vi "Control system.vi"() -> ()   [LabVIEW 2019]
panel:
  out "УЗ5":dbl
  out "Насос 8":bool=TRUE
  out "КР1":dbl
  out "КР7":dbl
  out "КР5":dbl
  out "КР3":dbl
  out "КР8":dbl
  out "КР4":dbl
  out "КР6":dbl
  out "КР2":dbl
  out "УЗ5":dbl
  out "УЗ7":dbl
  out "УЗ6":dbl
  out "СЧ2":dbl
  out "Манометр":dbl
  out "Насос 4":bool=TRUE
  out "ДМ2":dbl
  out "УЗ5":dbl
  out "Насос 3":bool=TRUE
  out "СЧ1":dbl
  out "УЗ2":dbl
  out "ДМ1":dbl
  out "УЗ3":dbl
  out "Объем подачи ДН2":dbl format="%#_13g"
  out "Донный клапан":bool=TRUE
  out "Дозирующий насос 2":bool=TRUE
  out "Насос 2":bool=TRUE
  out "PH1":dbl
  out "Насос 1":bool=TRUE
  out "УЗ2":dbl
  out "ДН1 объем подачи":dbl format="%#_13g"
  out "УЗ1":dbl
  out "Дозирующий насос 1":bool=TRUE
  out "УЗ4":dbl
  in  "Насос 8":bool=TRUE
  in  "КР1":dbl
  in  "КР8":dbl
  in  "КР4":dbl
  in  "КР7":dbl
  in  "КР6":dbl
  in  "КР5":dbl
  in  "КР3":dbl
  in  "КР2":dbl
  in  "Насос 4":bool=TRUE
  in  "Насос 3":bool=TRUE
  in  "объем подачи ДН2":dbl format="%#_13g"
  in  "Донный клапан":bool=TRUE
  in  "Дозирующий насос 2":bool=TRUE
  in  "Насос 2":bool=TRUE
  in  "ДН1 объем подачи":dbl format="%#_13g"
  in  "Дозирующий насос 1":bool=TRUE
  in  "Насос 1":bool=TRUE
  out "Статус работы":string
  in  "stop":bool
  # "Индикаторы промывки"
  # "Меабрана"
  # "Биореактор"
  # "II ступень очистки"
  # "I ступень очистки"
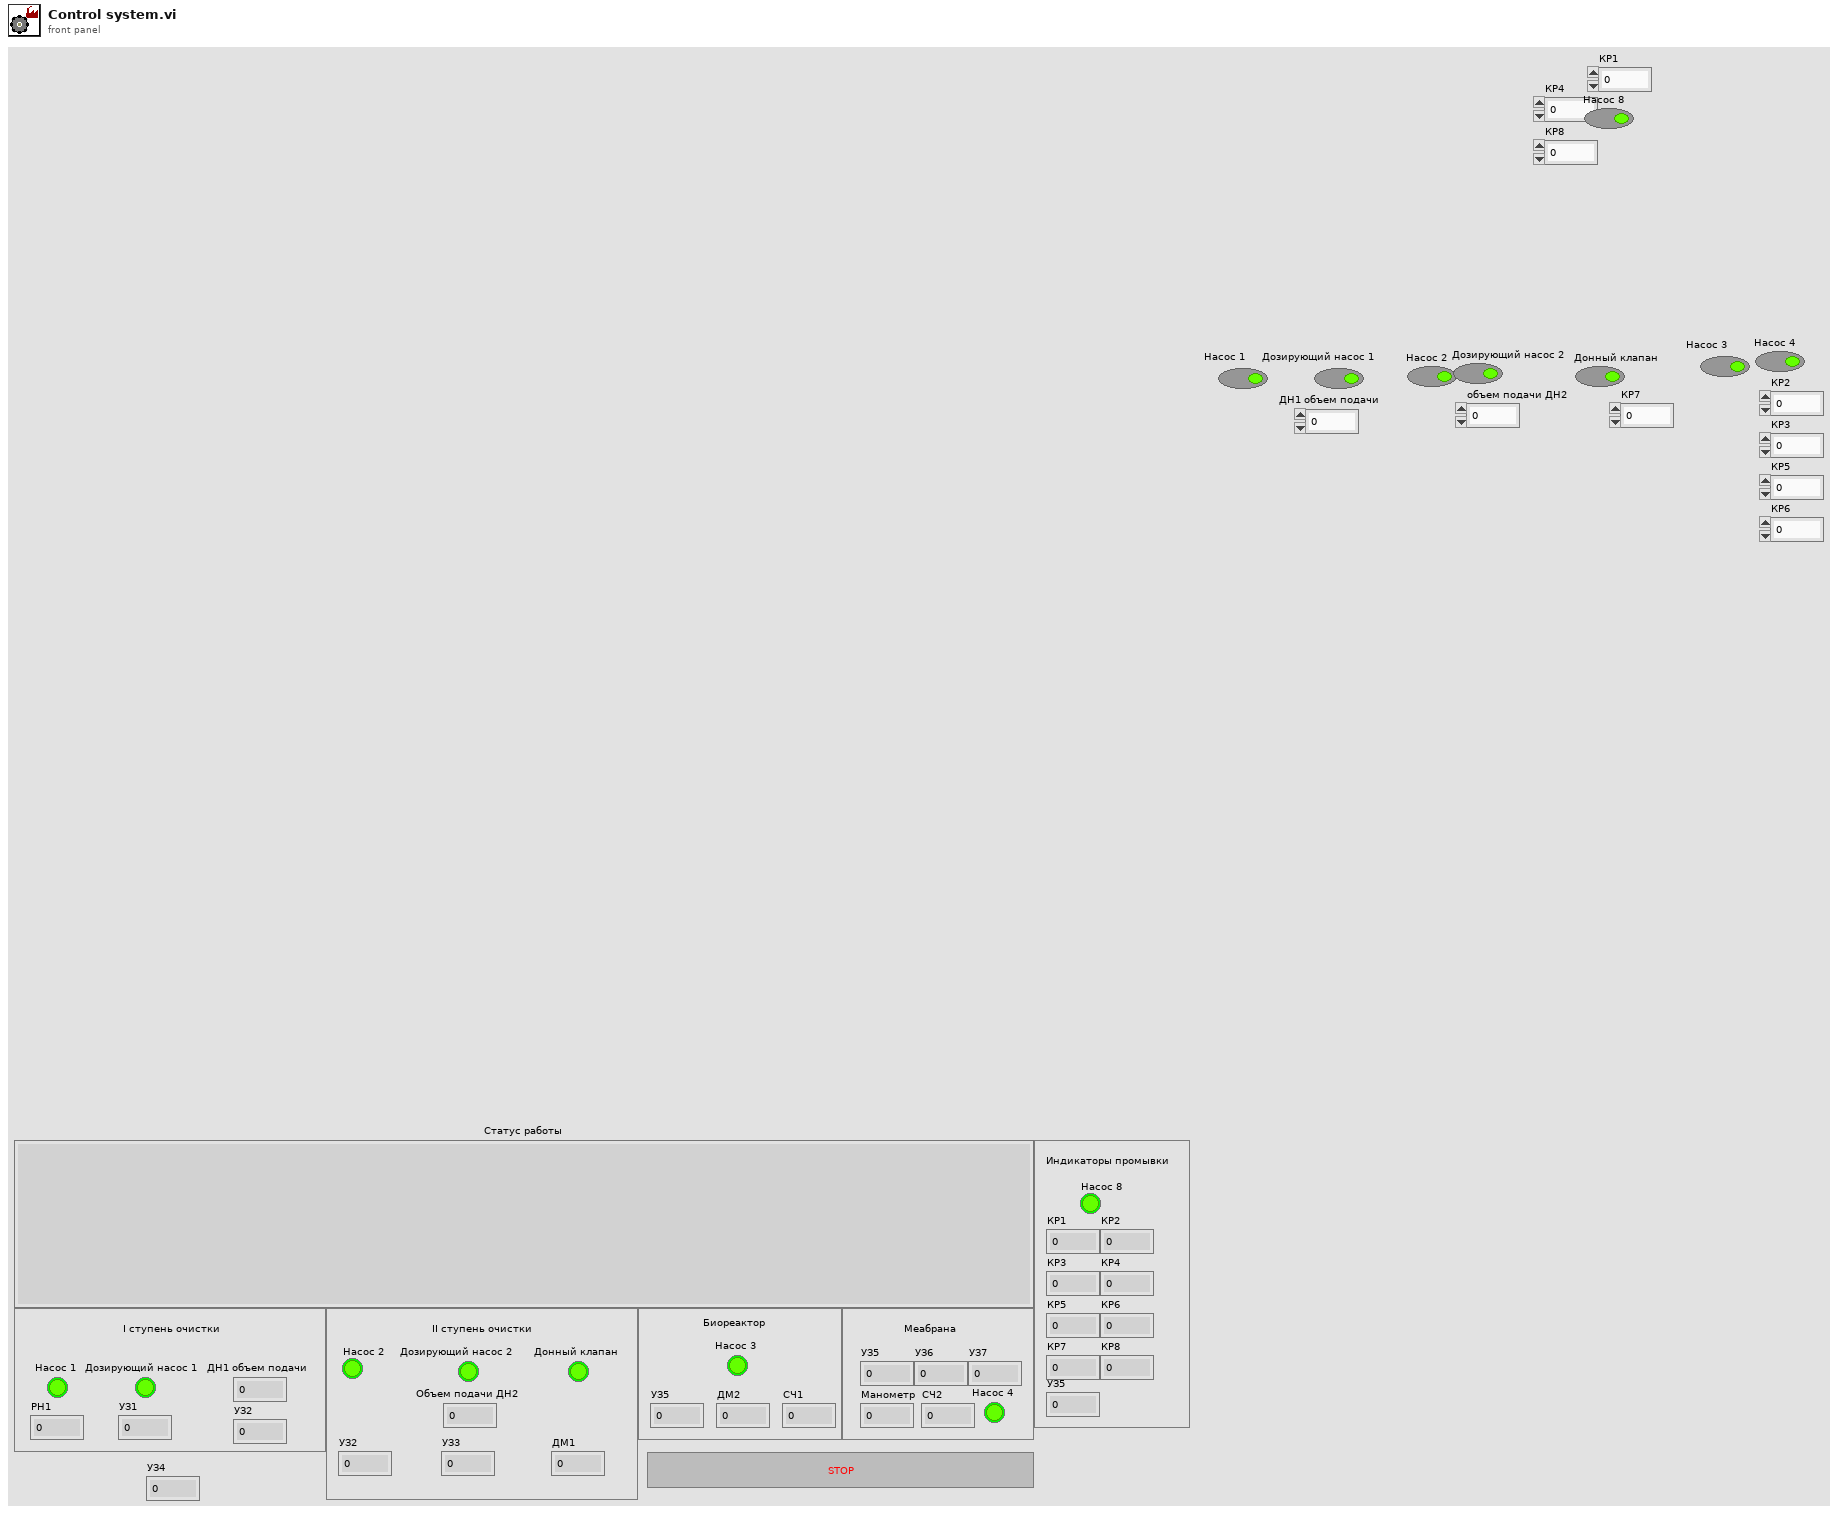
[diagram p1: front panel]
types:
  T1 = cluster{"УЗ1":dbl, "УЗ2":dbl, "УЗ3":dbl, "УЗ4":dbl, "УЗ5":dbl, "УЗ6":dbl, "УЗ7":dbl, "PH1":dbl, "ДМ1":dbl, "ДМ2":dbl, "Манометр":dbl, " СЧ1":dbl, " СЧ2":dbl}
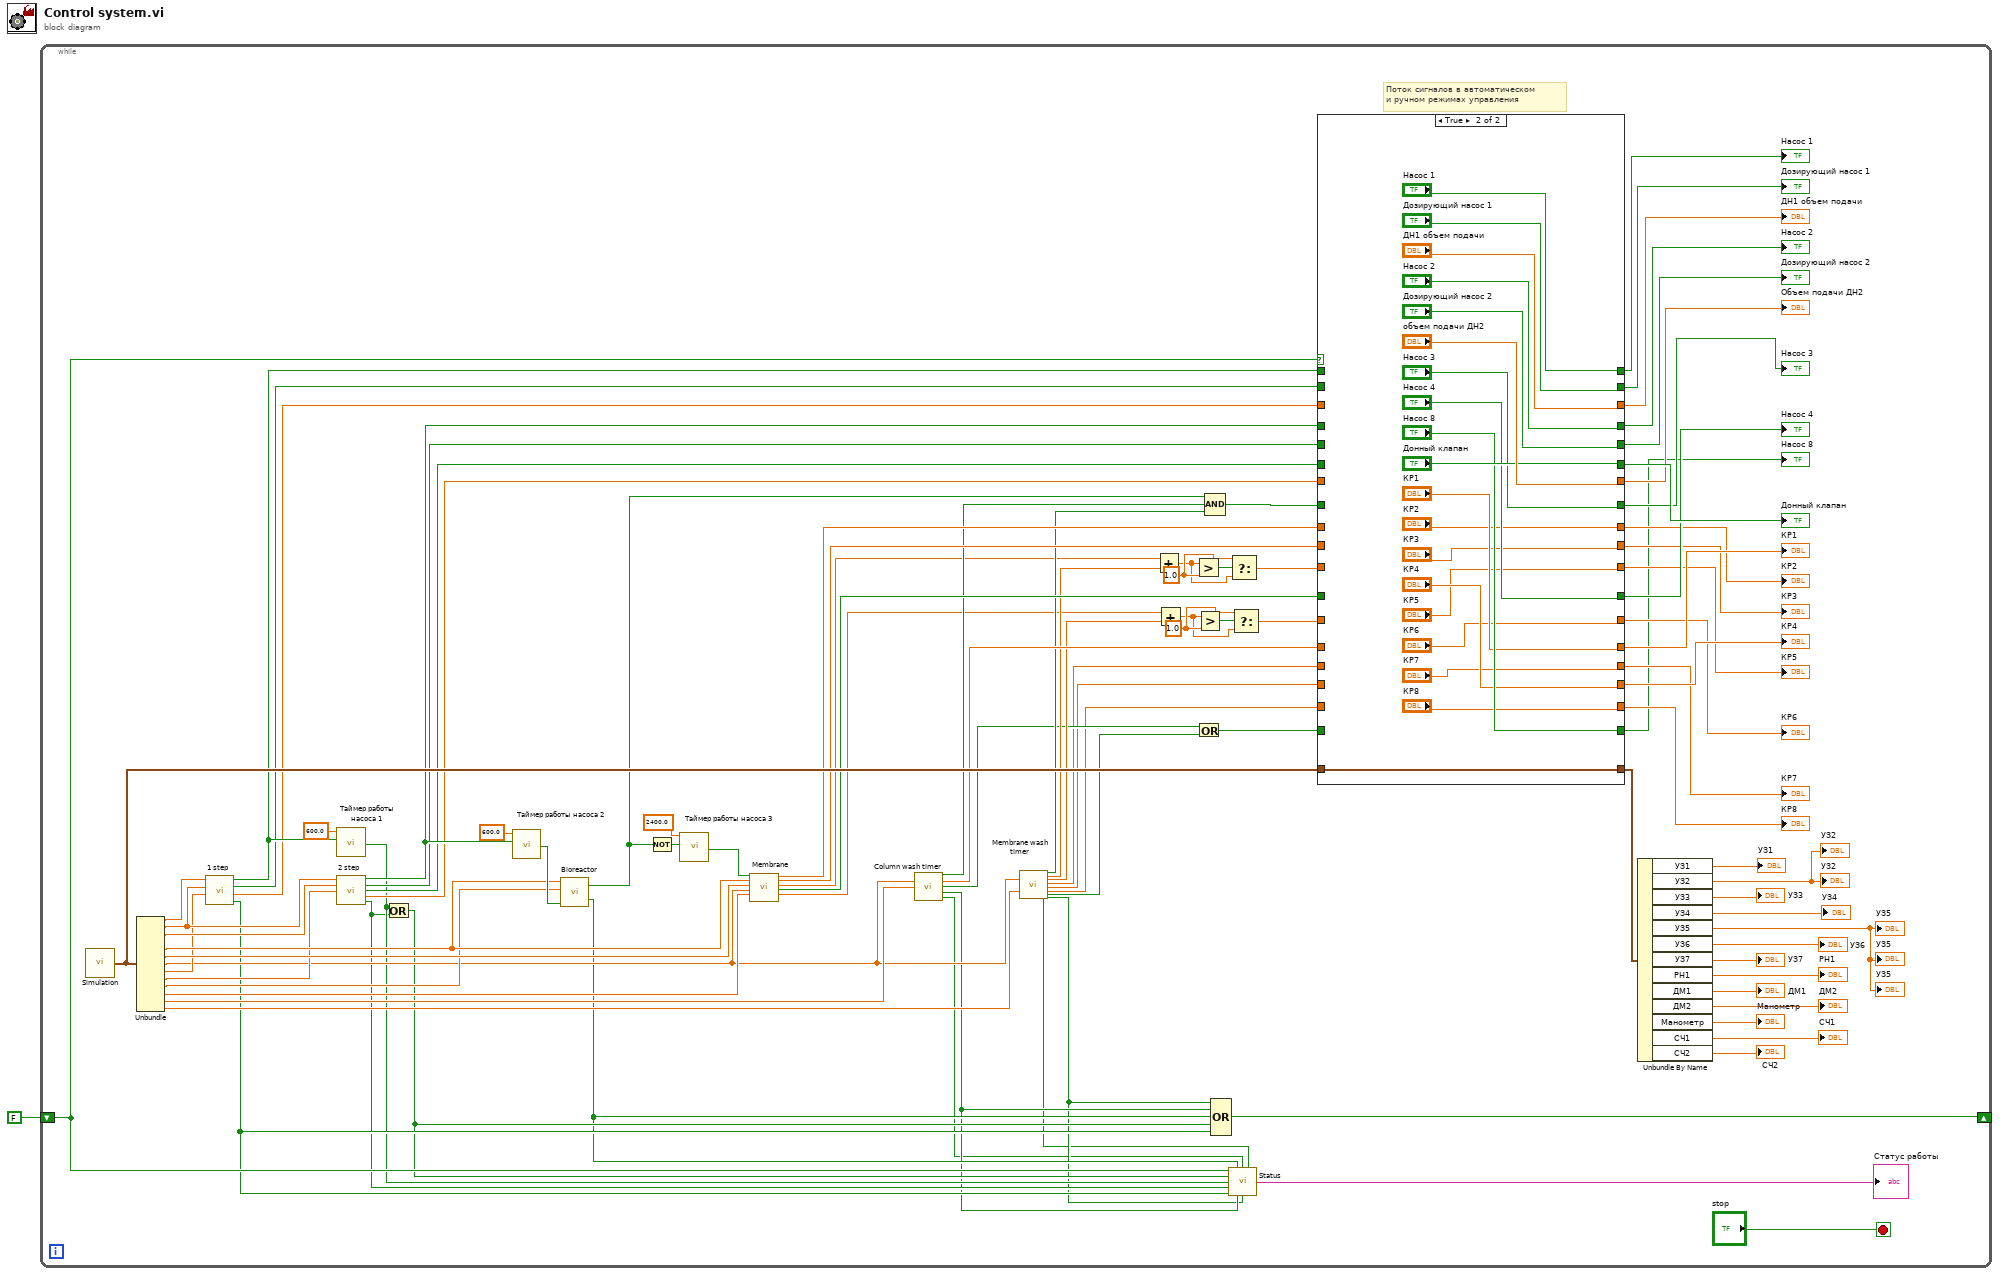
[diagram p0: block diagram]
diagram:
  n1 = while {
    shift-right: [w82] -> _
    shift-left: FALSE ("Error output") -> [w26]
    stop <- "stop" stop-if-true
    w55 = 1.0 ("y")
    w59 = 1.0 ("y")
    # "Поток сигналов в автоматическом \nи ручном режимах управления"
    n2 = call "Simulation.vi"() -> ("output cluster"=w80:T1)
    n3 = Unbundle(w80) -> ("УЗ1"=w92:dbl, "УЗ2"=w91:dbl, "УЗ3"=w90:dbl, "УЗ5"=w88:dbl, "УЗ6"=w89:dbl, "УЗ7"=w65:dbl, "PH1"=w87:dbl, "ДМ1"=w86:dbl, "ДМ2"=w85:dbl, "Манометр"=w84:dbl, "СЧ1"=w81:dbl, "СЧ2"=w64:dbl)  [unwired: 1 out]
    n4 = call "1 step.vi"("PH1"=w87, "УЗ2"=w91, "УЗ1"=w92) -> ("Error output"=w25:bool, "ДН1 объем подачи"=w77:dbl, "Дозирующий насос 1"=w78:bool, "Насос 1"=w79:bool)  [unwired: 1 in]
    n5 = call "Таймер работы насоса 1"("Time Target (s)"=600.0, "Reset"=w79) -> ("Time has Elapsed"=w23:bool)  [unwired: 10 in, 7 out]
    n6 = call "2 step.vi"("УЗ2"=w91, "УЗ3"=w90, "ДМ1"=w86) -> ("Насос 2"=w76:bool, "ДН2"=w75:bool, "Донный клапан"=w74:bool, "объем подачи ДН2"=w73:dbl, "Error output"=w22:bool)  [unwired: 8 in]
    n7 = Or(x=w23, y=w22) -> (x .or. y?=w24:bool)
    n8 = call "Таймер работы насоса 2"("Time Target (s)"=600.0, "Reset"=w76) -> ("Time has Elapsed"=w96:bool)  [unwired: 10 in, 7 out]
    n9 = call "Bioreactor.vi"("Timer"=w96, "ДМ2"=w85, "УЗ5"=w88) -> ("Error output"=w21:bool, "Насос 3"=w68:bool)  [unwired: 1 in]
    n10 = Not(x=w68) -> (.not. x?=w94:bool)
    n11 = call "Таймер работы насоса 3"("Time Target (s)"=2400.0, "Reset"=w94) -> ("Time has Elapsed"=w93:bool)  [unwired: 10 in, 7 out]
    n12 = call "Membrane.vi"("Насос 3"=w93, "УЗ5"=w88, "УЗ6"=w89, "УЗ7"=w65, "Манометр"=w84) -> ("КР2"=w72:dbl, "КР3"=w71:dbl, "КР5"=w61:dbl, "Насос 4"=w70:bool, "КР6"=w53:dbl)  [unwired: 10 in]
    n13 = call "Column wash timer.vi"("УЗ7"=w65, "СЧ1"=w81) -> ("Насос 3"=w67:bool, "КР1"=w66:dbl, "Насос 8"=w49:bool, "Error output"=w20:bool, "Status"=w17:bool)  [unwired: 9 in]
    n14 = call "Membrane wash timer.vi"("УЗ7"=w65, "СЧ2"=w64) -> ("Status"=w18:bool, "Насос 3"=w63:bool, "КР5"=w62:dbl, "КР6"=w52:dbl, "КР7"=w47:dbl, "КР4"=w46:dbl, "КР8"=w45:dbl, "Насос 8"=w48:bool, "Error output"=w19:bool)  [unwired: 17 in]
    n15 = Add(x=w61, y=w62) -> (x+y=w58:dbl)
    n16 = Add(x=w53, y=w52) -> (x+y=w54:dbl)
    n17 = Greater?(x=w58, y=w59) -> (0:w60:bool)
    n18 = Or(x=w49, y=w48) -> (x .or. y?=w50:bool)
    n19 = Greater?(x=w54, y=w55) -> (0:w56:bool)
    n20 = Compound Arithmetic op=AND(w68, w67, w63) -> (w69:bool)
    n21 = Compound Arithmetic op=OR(w19, w20, w21, w24, w25) -> (w82:bool)
    n22 = call "Status.vi"("Membrane washing status"=w18, "Column washing status"=w17, "Membrane washing error"=w19, "Bioreactor error"=w21, "Column washing error"=w20, "Error input"=w26, "2 step error"=w24, "2 step error-1"=w23, "2 step error-2"=w22, "1 step error"=w25) -> ("Status output"=→"Статус работы":string)  [unwired: 5 in]
    n23 = Select(t=w59, s=w60, f=w58) -> (s? t:f=w57:dbl)
    n24 = Select(t=w55, s=w56, f=w54) -> (s? t:f=w51:dbl)
    n25 = case shown="True" w26 {
      tunnel: w80 -> [w104 w136]
      tunnel: w79 -> [w117 _]
      tunnel: w78 -> [w116 _]
      tunnel: w77 -> [w115 _]
      tunnel: w76 -> [w114 _]
      tunnel: w75 -> [w113 _]
      tunnel: w74 -> [w112 _]
      tunnel: w73 -> [w111 _]
      tunnel: w69 -> [w110 _]
      tunnel: w72 -> [w109 _]
      tunnel: w71 -> [w108 _]
      tunnel: w57 -> [w107 _]
      tunnel: w70 -> [w106 _]
      tunnel: w51 -> [w105 _]
      tunnel: [w117 "Насос 1"] -> w44
      tunnel: [w116 "Дозирующий насос 1"] -> w43
      tunnel: [w115 "ДН1 объем подачи"] -> w42
      tunnel: [w114 "Насос 2"] -> w41
      tunnel: [w113 "Дозирующий насос 2"] -> w40
      tunnel: [w112 "Донный клапан"] -> w39
      tunnel: [w111 "объем подачи ДН2"] -> w38
      tunnel: [w110 "Насос 3"] -> w37
      tunnel: [w109 "КР2"] -> w34
      tunnel: [w108 "КР3"] -> w33
      tunnel: [w107 "КР5"] -> w31
      tunnel: [w106 "Насос 4"] -> w36
      tunnel: [w105 "КР6"] -> w30
      tunnel: [w104 w136] -> w15
      tunnel: w66 -> [w103 _]
      tunnel: w50 -> [w102 _]
      tunnel: [w103 "КР1"] -> w35
      tunnel: [w102 "Насос 8"] -> w27
      tunnel: w47 -> [w101 _]
      tunnel: w46 -> [w100 _]
      tunnel: w45 -> [w99 _]
      tunnel: [w101 "КР7"] -> w29
      tunnel: [w100 "КР4"] -> w32
      tunnel: [w99 "КР8"] -> w28
      frame False {
      }
      frame True {
      }
    }
    "Насос 1" <- w44
    "Дозирующий насос 1" <- w43
    "ДН1 объем подачи" <- w42
    "Насос 2" <- w41
    "Дозирующий насос 2" <- w40
    "Донный клапан" <- w39
    "Объем подачи ДН2" <- w38
    "Насос 4" <- w36
    "КР2" <- w34
    "КР3" <- w33
    "КР5" <- w31
    "КР6" <- w30
    "КР7" <- w29
    "КР4" <- w32
    "КР8" <- w28
    "КР1" <- w35
    "Насос 8" <- w27
    "Насос 3" <- w37
    n26 = Unbundle By Name(w15) -> ("УЗ1"=→"УЗ1":dbl, "УЗ2"=→"УЗ2" →"УЗ2":dbl, "УЗ3"=→"УЗ3":dbl, "УЗ4"=→"УЗ4":dbl, "УЗ5"=→"УЗ5" →"УЗ5" →"УЗ5":dbl, "УЗ6"=→"УЗ6":dbl, "УЗ7"=→"УЗ7":dbl, "PH1"=→"PH1":dbl, "ДМ1"=→"ДМ1":dbl, "ДМ2"=→"ДМ2":dbl, "Манометр"=→"Манометр":dbl, "СЧ1"=→"СЧ1":dbl, "СЧ2"=→"СЧ2":dbl)
  }
